vi "Write age.vi"(8 "error in (no error)":errorcluster, 10 "age":dbl, 11 "myClass in":refnum<class "myClass.lvclass">) -> (0 "error out":errorcluster, 3 "myClass out":refnum<class "myClass.lvclass">)   [LabVIEW 2013, in "myClass.lvclass"]
uses:
  myClass.lvclass
  myClass.lvclass/myClass.ctl
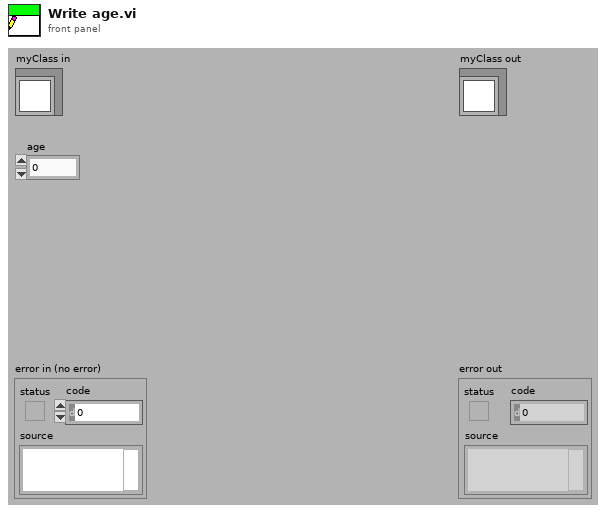
[diagram p1: front panel]
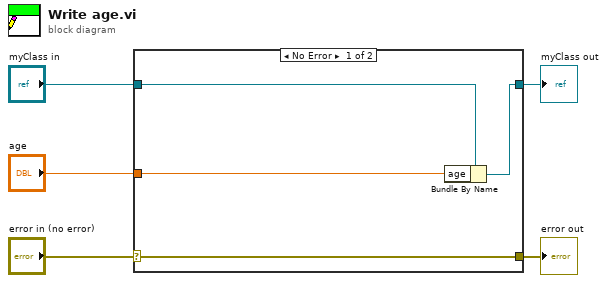
[diagram p0: block diagram]
diagram:
  n1 = case shown="No Error" "error in (no error)" {
    selector: "error in (no error)" -> [w9 w10]
    tunnel: [w9 w10] -> w4
    tunnel: [w7 w11] -> w2
    tunnel: "myClass in" -> [w8 w11]
    tunnel: "age" -> [w6 _]
    frame No Error {
      n2 = Bundle By Name(cluster=w8, "age"=w6) -> (w7:refnum<class "myClass.lvclass">)
    }
    frame Error {
    }
  }
  "error out" <- w4
  "myClass out" <- w2
